vi "test.vi"   [LabVIEW 2019, in "Database Viewer.lvclass"]
uses:
  Database Viewer.lvclass
  <userlib>/LevyLab/LV-Data/LV-Data.PG/LV-Data.PGSQL.lvclass
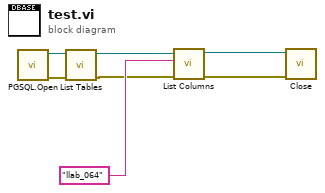
[diagram p0: block diagram]
diagram:
  n1 = call <userlib>:"PGSQL.Open.vi"() -> ("error out"=w7:errorcluster, "Data.PG out"=w6:refnum<class "LV-Data.PGSQL.lvclass">)  [unwired: 10 in]
  n2 = call <userlib>:"List Tables.vi"("error in (no error)"=w7, "Data.PG"=w6) -> ("error out"=w4:errorcluster, "Data.PG"=w3:refnum<class "LV-Data.PGSQL.lvclass">)  [unwired: 6 in, 2 out]
  n3 = call <userlib>:"List Columns.vi"("error in (no error)"=w4, "Table Path"="llab_064", "Data.PG"=w3) -> ("error out"=w2:errorcluster, "Data.PG out"=w1:refnum<class "LV-Data.PGSQL.lvclass">)  [unwired: 4 in, 3 out]
  n4 = call-dynamic "Close.vi"("error in (no error)"=w2, "Data.PG in"=w1) -> ()  [unwired: 8 in, 2 out]
